vi "Get state.vi"(6 "wait for reply (T)":bool=TRUE, 8 "error in":errorcluster, 10 "Address":u8, 11 "Module ID":i32=-1) -> (0 "error out":errorcluster, 1 "timed out?":bool, 3 "Device state":T1=enum."Configuration")   [LabVIEW 2020, in "FCR100.lvlib"]
doc: "Request to get error and controller state (xxTS).\n_____\nCreated using DQMH Event Scripter 6.1.0.128."
uses:
  FCR100.lvlib
  Get state Argument--cluster.ctl
  Get state (Reply Payload)--cluster.ctl
  Support/Device state -- enum.ctl
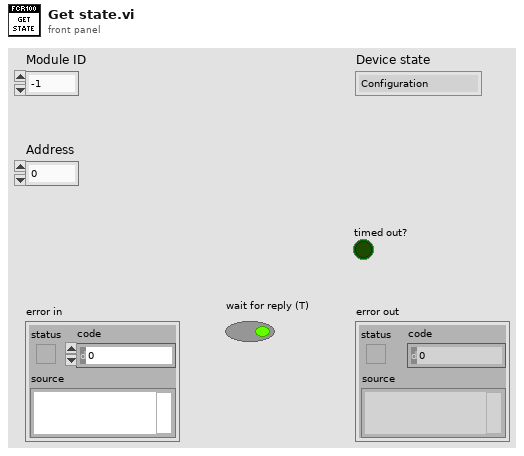
[diagram p1: front panel]
types:
  T1 = typedef "FCR100.lvlib/Device state -- enum.ctl" = enum16{"Not referenced", "Configuration", "Disable", "Ready", "Homing", "Motion"}
  T2 = typedef "FCR100.lvlib/Get state Argument--cluster.ctl" = cluster{"Module ID":i32, "Address":u8, "Wait Notifier":refnum<notifier>, "wait for reply":bool}
  T3 = typedef "FCR100.lvlib/Request Events--cluster.ctl" = cluster{"Stop Module":refnum<user-event>, "Show Panel":refnum<user-event>, "Hide Panel":refnum<user-event>, "Show Diagram":refnum<user-event>, "Get Module Execution Status":refnum<user-event>, "Connect with dialog":refnum<user-event>, "Change configuration state":refnum<user-event>, "Change disable state":refnum<user-event>, "Search Home":refnum<user-event>, "Stop movement":refnum<user-event>, "Get state":refnum<user-event>, "Set acceleration":refnum<user-event>, "Get acceleration":refnum<user-event>, "Set velocity":refnum<user-event>, "Get velocity":refnum<user-event>, "Get ETA":refnum<user-event>, "Move absolute":refnum<user-event>, "Move relative":refnum<user-event>, "Get current position":refnum<user-event>}
  T4 = typedef "FCR100.lvlib/Get state (Reply Payload)--cluster.ctl" = cluster{"Device state":T1, "error":errorcluster}
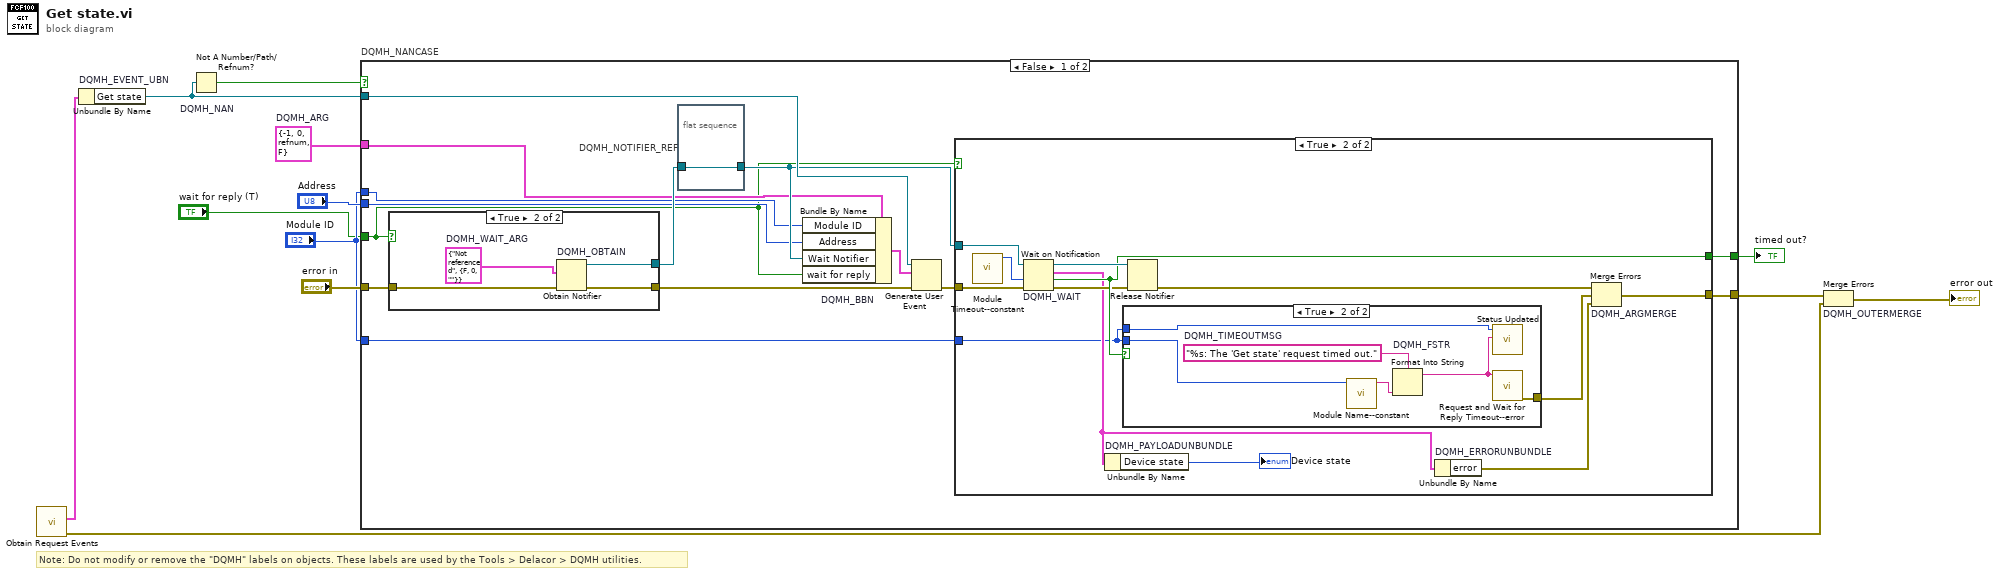
[diagram p0: block diagram]
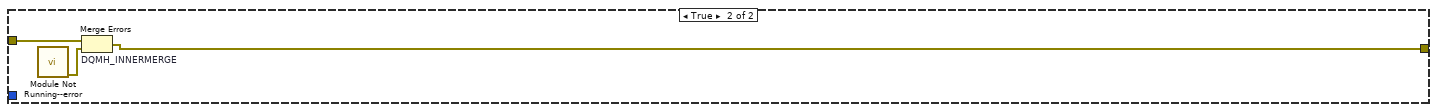
[diagram p5: hidden frame]
diagram:
  w6 = T2 {"Module ID"=-1, "Address"=0, "Wait Notifier"=refnum, "wait for reply"=FALSE}  # DQMH_ARG
  # "Note: Do not modify or remove the \"DQMH\" labels on objects. These labels are used by the Tools > Delacor > DQMH utilities."
  n1 = call "Obtain Request Events.vi"() -> ("error out"=w2:errorcluster, "FCR100 Request Events"=w1:T3)  [unwired: 10 in]
  n2 = Unbundle By Name "DQMH_EVENT_UBN"(w1) -> ("Get state"=w10:refnum<user-event>)
  n3 = Not A Number/Path/Refnum? "DQMH_NAN"(number/path/refnum=w10) -> (NaN/Path/Refnum?=w9:bool)
  n4 = case "DQMH_NANCASE" shown="False" w9 {
    tunnel: "error in" -> [w26 w55]
    tunnel: w10 -> [w24 _]
    tunnel: [w21 w54] -> w7
    tunnel: [w22 _] -> w8
    tunnel: w6 -> [w17 _]
    tunnel: "Module ID" -> [w16 _]
    tunnel: "Address" -> [w15 _]
    tunnel: "Module ID" -> [w14 _]
    tunnel: "wait for reply (T)" -> [w13 _]
    frame False {
      n5 = case shown="True" w13 {
        tunnel: w26 -> [w48 w52]
        tunnel: [w48 w51] -> w23
        tunnel: [_ w49] -> w19
        frame False {
        }
        frame True {
          w50 = T4 {"Device state"=enum."Not referenced", "error"={"status"=FALSE, "code"=0, "source"=""}}  # DQMH_WAIT_ARG
          n6 = Obtain Notifier "DQMH_OBTAIN"(notification data type=w50, error in (no error)=w52) -> (notifier out=w49:refnum<notifier>, error out=w51:errorcluster)  [unwired: 2 in, 1 out]
        }
      }
      n7 = flat-sequence "DQMH_NOTIFIER_REF" {
        tunnel: w19 -> [w27]
        tunnel: [w27] -> w18
        frame #0 {
        }
      }
      n8 = Bundle By Name "DQMH_BBN"(cluster=w17, "Module ID"=w16, "Address"=w15, "Wait Notifier"=w18, "wait for reply"=w13) -> (w20:T2)
      n9 = Generate User Event(user event=w24, event data cluster=w20, error in=w23) -> (error out=w25:errorcluster)  [unwired: 1 in, 1 out]
      n10 = case shown="True" w13 {
        tunnel: w25 -> [w28 w41]
        tunnel: w18 -> [_ w40]
        tunnel: [_ w38] -> w22
        tunnel: [w28 w37] -> w21
        tunnel: w14 -> [_ w30]
        frame False {
        }
        frame True {
          n11 = call "Module Timeout--constant.vi"() -> ("Module Timeout"=w31:i32)  [unwired: 11 in]
          n12 = Wait on Notification "DQMH_WAIT"(notifier=w40, timeout in ms (-1)=w31, error in (no error)=w41) -> (notifier out=w39:refnum<notifier>, notification=w32:T4, timed out?=w38:bool, error out=w36:errorcluster)  [unwired: 1 in]
          n13 = Unbundle By Name "DQMH_PAYLOADUNBUNDLE"(w32) -> ("Device state"=→"Device state":T1)
          n14 = case shown="True" w38 {
            tunnel: [_ w45] -> w33
            tunnel: w30 -> [_ w43]
            tunnel: w30 -> [_ w42]
            frame False {
            }
            frame True {
              w47 = "%s: The 'Get state' request timed out."  # DQMH_TIMEOUTMSG
              n15 = call "Module Name--constant.vi"("Module ID"=w42) -> ("Module Name"=w44:string)  [unwired: 10 in]
              n16 = Format Into String "DQMH_FSTR"(format string=w47, w44) -> (resulting string=w46:string)  [unwired: 2 in, 1 out]
              n17 = call "Status Updated.vi"("Status"=w46, "Module ID"=w43) -> ()  [unwired: 9 in, 1 out]
              n18 = call "Request and Wait for Reply Timeout--error.vi"("Error Message"=w46) -> ("error out"=w45:errorcluster)  [unwired: 10 in]
            }
          }
          n19 = Release Notifier(notifier=w39, error in (no error)=w36) -> (error out=w35:errorcluster)  [unwired: 1 in, 2 out]
          n20 = Unbundle By Name "DQMH_ERRORUNBUNDLE"(w32) -> ("error"=w34:errorcluster)
          n21 = Merge Errors "DQMH_ARGMERGE"(w35, w33, w34) -> (w37:errorcluster)
        }
      }
    }
    frame True {
      n22 = call "Module Not Running--error.vi"() -> ("error out"=w53:errorcluster)  [unwired: 11 in]
      n23 = Merge Errors "DQMH_INNERMERGE"(w55, w53) -> (w54:errorcluster)
    }
  }
  "timed out?" <- w8
  n24 = Merge Errors "DQMH_OUTERMERGE"(w7, w2) -> (→"error out":errorcluster)
